vi "VI Tree.vi"   [LabVIEW 2012, in "Phidget Sound Sensor.lvlib"]
doc: "This is the instrument driver for the Phidget Light Sensor. The VI Tree displays all the user-callable VIs of the instrument driver in an organized table."
uses:
  <instrlib>/Phidgets/Phidget Sound Sensor/Phidget Sound Sensor.lvlib
  <instrlib>/Phidgets/Phidget Sound Sensor/Public/SoundSensorStart.vi
  <instrlib>/Phidgets/Phidget Sound Sensor/Public/SoundSensorOpen.vi
  <instrlib>/Phidgets/Phidget Sound Sensor/Public/SoundSensorClose.vi
panel:
  # "(c) 2015 Phidgets Inc..  ALL RIGHTS RESERVED."
  # "SEE DIAGRAM\nFOR VI TREE."
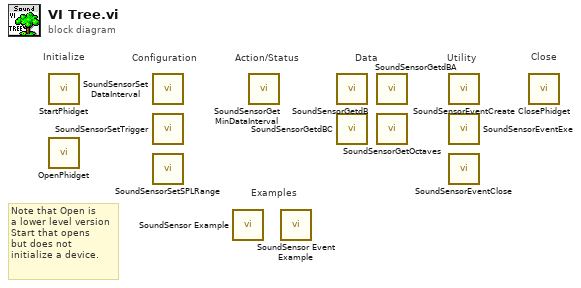
[diagram p0: block diagram]
diagram:
  # "Note that Open is\na lower level version\nStart that opens\nbut does not \ninitialize a device."
  # "Examples"
  # "Configuration"
  # "Utility"
  # "Data"
  # "Action/Status"
  # "Close"
  # "Initialize"
  n1 = call-poly <instrlib>:"StartPhidget.vi"() -> ()  [unwired: 12 in, 4 out]
  n2 = call-poly <instrlib>:"OpenPhidget.vi"() -> ()  [unwired: 8 in, 4 out]
  n3 = call <instrlib>:"SoundSensorSetDataInterval.vi"() -> ()  [unwired: 9 in, 2 out]
  n4 = call <instrlib>:"SoundSensorSetTrigger.vi"() -> ()  [unwired: 9 in, 2 out]
  n5 = call <instrlib>:"SoundSensorSetSPLRange.vi"() -> ()  [unwired: 9 in, 2 out]
  n6 = call <instrlib>:"SoundSensor Example.vi"() -> ()  [unwired: 12 in]
  n7 = call <instrlib>:"SoundSensorGetMinDataInterval.vi"() -> ()  [unwired: 8 in, 3 out]
  n8 = call <instrlib>:"SoundSensor Event Example.vi"() -> ()  [unwired: 12 in]
  n9 = call <instrlib>:"SoundSensorGetdB.vi"() -> ()  [unwired: 8 in, 3 out]
  n10 = call <instrlib>:"SoundSensorGetdBC.vi"() -> ()  [unwired: 8 in, 3 out]
  n11 = call <instrlib>:"SoundSensorGetdBA.vi"() -> ()  [unwired: 8 in, 3 out]
  n12 = call <instrlib>:"SoundSensorGetOctaves.vi"() -> ()  [unwired: 8 in, 3 out]
  n13 = call <instrlib>:"SoundSensorEventCreate.vi"() -> ()  [unwired: 9 in, 3 out]
  n14 = call <instrlib>:"SoundSensorEventExe.vi"() -> ()  [unwired: 10 in, 10 out]
  n15 = call <instrlib>:"SoundSensorEventClose.vi"() -> ()  [unwired: 10 in, 2 out]
  n16 = call-poly <instrlib>:"ClosePhidget.vi"() -> ()  [unwired: 11 in, 1 out]
